vi "Subpanel Call.vi"(8 "error in (no error)":errorcluster) -> (0 "error out":errorcluster)   [LabVIEW 2013]
uses:
  Global Variables/gl_UI Ctrl Refs.vi
  Global Variables/gl_Subpanel VI ref.vi
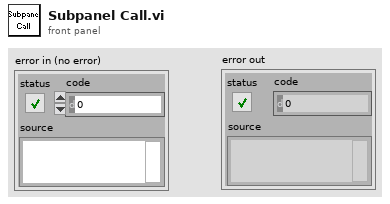
[diagram p1: front panel]
types:
  T1 = typedef "UI ctrl refs cluster.ctl" = cluster{"Top level VI path":path, "Top level VI ref":refnum<vi>, "User menu ref":refnum<k9>, "Sub Panel control":refnum<vi>, "Imaging Param Tab":refnum<vi>, "Occurrence-Start drivers":refnum<k4>, "Occurrence-Speed logging initialised":refnum<k4>, "Occurrence-XYZ stage initialised":refnum<k4>, "Exit button":refnum<vi>, "Status ind":refnum<vi>, "Return to Origin":refnum<vi>, "Speed Logging":refnum<vi>, "Time Lapse":refnum<vi>, "Live Imaging":refnum<vi>, "AOL Z Stack":refnum<vi>, "Motor Z Stack":refnum<vi>, "Funct Acq button":refnum<vi>, "Hard Shutter":refnum<vi>, "Virtual Shutter":refnum<vi>, "Laser Power":refnum<vi>, "AOL Mode":refnum<vi>, "Frame Size":refnum<vi>, "Field of View":refnum<vi>, "Dwell Time":refnum<vi>, "Zoom":refnum<vi>, "AOL Z":refnum<vi>, "Objective":refnum<vi>, "Axis":refnum<vi>, "Paths & Names":refnum<vi>, "Experiment folder path (ind.)":refnum<vi>, "Last State (Ind.)":refnum<vi>, "Laser wavelength ind (nm)":refnum<vi>, "Averages":refnum<vi>, "Angle (degrees)":refnum<vi>, "X centre":refnum<vi>, "Y centre":refnum<vi>, "Plane Mode":refnum<vi>, "# Planes":refnum<vi>, "Z Start":refnum<vi>, "Z Stop":refnum<vi>, "Z Step":refnum<vi>, "PMT 1":refnum<vi>, "PMT 2":refnum<vi>, "Stage XYZ Position":refnum<vi>, "Pockels@Z Start":refnum<vi>, "Pockels@Z Stop":refnum<vi>, "Obtain Z Start":refnum<vi>, "Obtain Z Stop":refnum<vi>, "Live stim.trig.period":refnum<vi>, "Live stim.trig.enable":refnum<vi>, "Funct. Acq. Pockels Modulation":refnum<vi>, "Enable Video Recording":refnum<vi>, "Video Record-Live Imaging":refnum<vi>, "Video Record-Funct acq":refnum<vi>, "AOL Z-stack Chirps Ready (ind)":refnum<vi>, "Center freq ind (nm)":refnum<vi>, "Logging queue (ind)":refnum<vi>, "Back aperture power (ind.)":refnum<vi>, "Power after objective (ind.)":refnum<vi>, "Switch user":refnum<vi>}
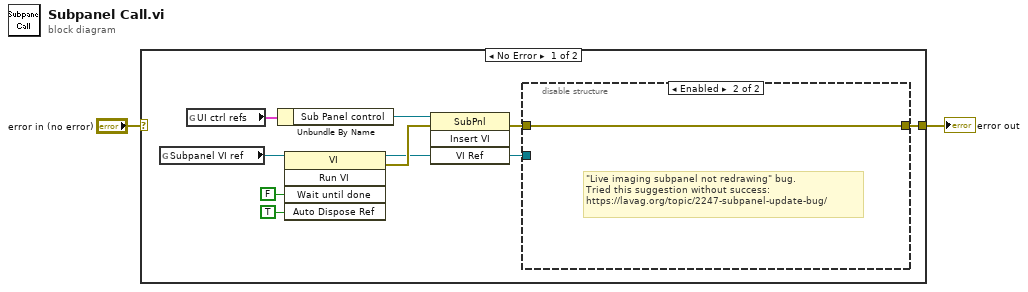
[diagram p0: block diagram]
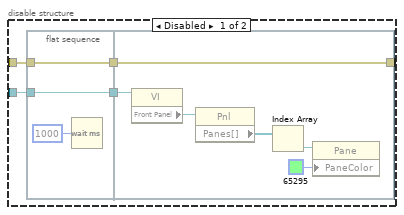
[diagram p2: hidden frame]
diagram:
  n1 = case shown="No Error" "error in (no error)" {
    selector: "error in (no error)" -> [_ w27]
    tunnel: [w3 w27] -> w1
    frame No Error {
      n2 = global read "gl_Subpanel VI ref.vi" "Subpanel VI ref"() -> (w6:refnum<vi>)
      n3 = global read "gl_UI Ctrl Refs.vi" "UI ctrl refs"() -> (w7:T1)
      n4 = Unbundle By Name(w7) -> ("Sub Panel control"=w10:refnum<vi>)
      n5 = invoke on="Invoke Node" class="VI" method="Run VI"(reference=w6, "Wait until done"=FALSE ("Wait Until Done"), "Auto Dispose Ref"=TRUE ("Auto Dispose Reference")) -> (reference out=w5:refnum<vi>, error out=w9:errorcluster)  [unwired: 2 in, 3 out]
      n6 = invoke on="Invoke Node" class="SubPnl" method="Insert VI"(reference=w10, error in=w9, "VI Ref"=w5) -> (error out=w4:errorcluster)  [unwired: 1 in, 3 out]
      n7 = disable-structure shown="Enabled" {
        disable-tunnel: w5 -> [w14 _]
        disable-tunnel: w4 -> [w13 w26]
        disable-tunnel: [w12 w26] -> w3
        frame Disabled {
          n8 = flat-sequence {
            tunnel: w13 -> [w18]
            tunnel: w14 -> [w19]
            tunnel: [w19] -> w16
            tunnel: [w18] -> w15
            tunnel: [w20] -> w12
            tunnel: w16 -> [w21]
            tunnel: w15 -> [w20]
            frame #0 {
              n9 = Wait (ms)(milliseconds to wait=u32 1000) -> ()  [unwired: 1 out]
            }
            frame #1 {
              n10 = property class="VI"(reference=w21) -> ("Front Panel"=w22:refnum<vi>)  [unwired: 1 in, 2 out]
              n11 = property class="Pnl"(reference=w22) -> ("Panes[]"=w23:refnum<vi>[])  [unwired: 1 in, 2 out]
              n12 = Index Array(array=w23) -> (element=w24:refnum<vi>)  [unwired: 1 in]
              n13 = property class="Pane"(reference=w24, "PaneColor"=u32 65295 ("Color")) -> ()  [unwired: 1 in, 2 out]
            }
          }
        }
        frame Enabled {
          # "\"Live imaging subpanel not redrawing\" bug.\nTried this suggestion without success: \nhttps://lavag.org/topic/2247-subpanel-update-bug/"
        }
      }
    }
    frame Error {
    }
  }
  "error out" <- w1
